vi "Telnet_RW_wResp_noLog.vi"(5 "timeout ms":i32=500, 6 "bytes to read (1024)":i32=1024, 7 "Delay Time (s)":dbl=0.3, 8 "error in (no error)":errorcluster, 9 "expected string":string, 10 "Write Telnet Command":string, 11 "connection ID":refnum<k5>) -> (0 "error out":errorcluster, 1 "String found?":bool, 2 "string out":string, 3 "connection ID out":refnum<k5>)   [LabVIEW 2018]
doc: "This VI sends a command using telnet and verifies the response is the expected one."
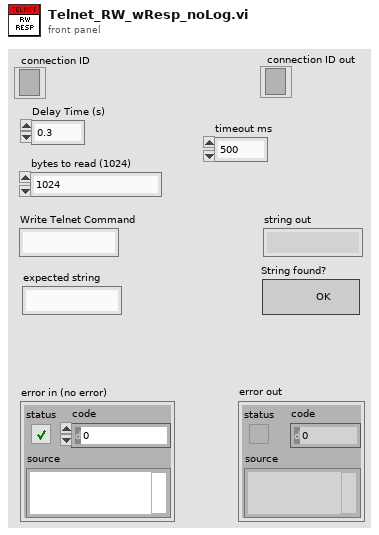
[diagram p1: front panel]
types:
  T1 = enum16{"Standard", "Buffered", "CRLF", "Immediate"}
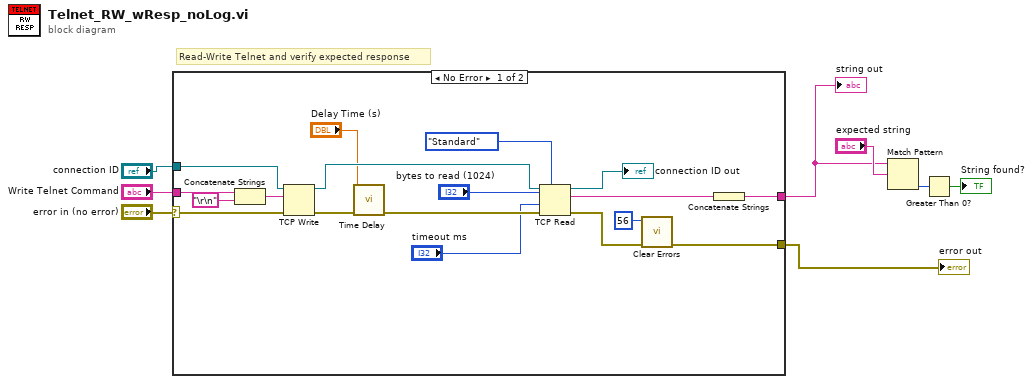
[diagram p0: block diagram]
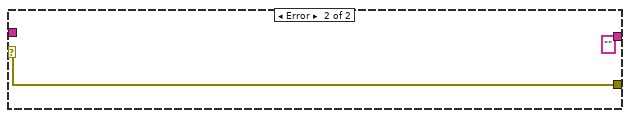
[diagram p2: hidden frame]
diagram:
  # "Read-Write Telnet and verify expected response"
  n1 = case shown="No Error" "error in (no error)" {
    selector: "error in (no error)" -> [w11 w27]
    tunnel: [w19 ""] -> w2
    tunnel: [w18 w27] -> w1
    tunnel: "Write Telnet Command" -> [w15 _]
    tunnel: "connection ID" -> [w12 _]
    frame No Error {
      n2 = Concatenate Strings(w15, "\r\n") -> (w17:string)
      n3 = TCP Write(connection ID=w12, data in=w17, error in (no error)=w11) -> (connection ID out=w14:refnum<k5>, error out=w13:errorcluster)  [unwired: 1 in, 1 out]
      n4 = call "Time Delay"("error in (no error)"=w13, "Delay Time (s)"="Delay Time (s)") -> ("error out"=w21:errorcluster)  [unwired: 9 in]
      n5 = TCP Read(connection ID=w14, bytes to read="bytes to read (1024)", error in (no error)=w21, 7:T1."Standard" ("mode (standard)"), 9:"timeout ms") -> (connection ID out=→"connection ID out":refnum<k5>, data out=w20:string, error out=w23:errorcluster)
      n6 = call "Clear Errors.vi"("error in (no error)"=w23, "specific error code to clear (0: all)"=56) -> ("error out"=w18:errorcluster)  [unwired: 4 in, 1 out]
      n7 = Concatenate Strings(w20) -> (w19:string)
    }
    frame Error {
    }
  }
  "string out" <- w2
  "error out" <- w1
  n8 = Match Pattern(string=w2, regular expression="expected string") -> (offset past match=w5:i32)  [unwired: 1 in, 3 out]
  n9 = Greater Than 0?(x=w5) -> (x > 0?=→"String found?":bool)
